vi "Write Status.vi"(8 "error in (no error)":errorcluster, 10 "Status":string, 11 "VisualizeBase_class in":refnum<class "VisualizeBase.lvclass">) -> (0 "error out":errorcluster, 3 "VisualizeBase_class out":refnum<class "VisualizeBase.lvclass">)   [LabVIEW 2018, in "Visualization.lvlib" / "VisualizeBase.lvclass"]
uses:
  VisualizeBase.lvclass
  VisualizeBase.lvclass/VisualizeBase.ctl
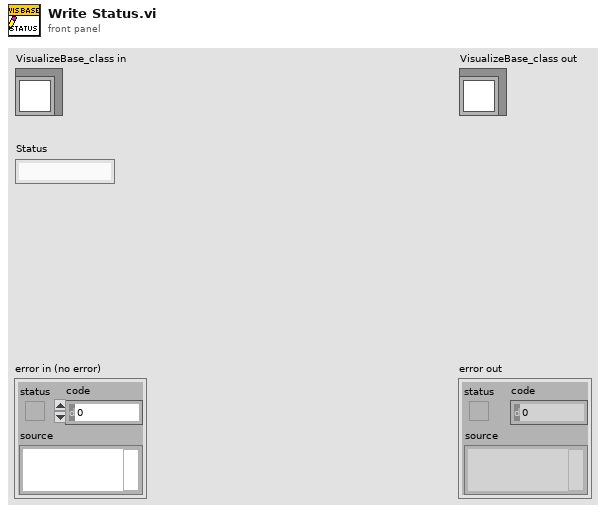
[diagram p1: front panel]
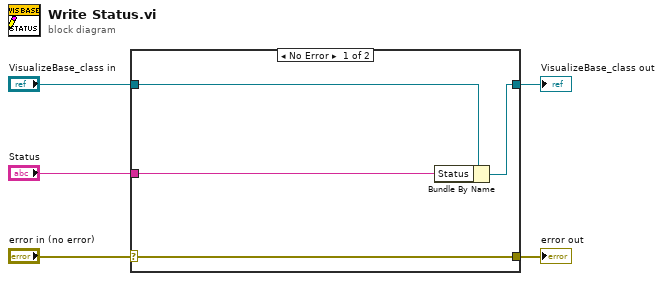
[diagram p0: block diagram]
diagram:
  n1 = case shown="No Error" "error in (no error)" {
    selector: "error in (no error)" -> [w9 w10]
    tunnel: [w9 w10] -> w4
    tunnel: [w7 w11] -> w2
    tunnel: "VisualizeBase_class in" -> [w8 w11]
    tunnel: "Status" -> [w6 _]
    frame No Error {
      n2 = Bundle By Name(cluster=w8, "Status"=w6) -> (w7:refnum<class "VisualizeBase.lvclass">)
    }
    frame Error {
    }
  }
  "error out" <- w4
  "VisualizeBase_class out" <- w2
